vi "Live Capture Functional Stack2.vi"() -> ()   [LabVIEW 2014]
uses:
  subvis/Stack Track.ctl
  subvis/Stack_State.ctl
panel:
  out "error out 2":errorcluster {"code" format="%.0x"}
  out "Count":i32
  in  "Temp":path=path "C:/temp.tmp"
  in  "Frames":i32=100
  in  "HardDisk Record":bool
  in  "Internal Line Interval":dbl
  in  "Slit Width / Lines":sgl=150.0
  in  "Camera Readout Mode":u16(ring)=12 items=["Full Frame"=1, "Slit Scanning"=12]
  in  "Readout Direction":sgl(ring)=1.0 items=["Forward"=1, "Backward"=2]
  in  "Trigger Mode":sgl(ring)=1.0 items=["Normal"=1, "Start "=6]
  in  "Trigger Source":sgl(ring)=2.0 items=["Internal"=1, "External"=2]
  out "Enum":T1
  out "Image":u16[][](graph)
  out "Saving":bool
  in  "AutoIncrement":bool=TRUE
  in  "Path":path=path "C:/Users/spim/Desktop/Craig Cap/temp/a.tiff"
  in  "Frames":i32=100
  out "Frame Index":i32
  out "error out":errorcluster
  in  "stop":bool
  in  "Capture":bool
  out "Total Frames":i32
  out "Elapsed Time":u32
  out "Software FPS":dbl
  out "Camera FPS":dbl
  in  "H Offset":i32 min=0 max=0 step=4
  in  "H Width":i32 min=0 max=2048 step=4
  out "SMD":dbl
  out "SHO":i32
  in  "V Offset":i32 min=0 max=0 step=4
  in  "V Width":i32 min=0 max=2048 step=4
  in  "Binning":u16(ring) items=["1x1"=1, "2x2"=2, "4x4"=4]
  out "SHW":i32
  out "SVO":i32
  out "SVW":i32
  in  "Scan Mode":dbl min=0.0 max=2.0 step=1.0
  in  "Exposure":dbl min=0.0 max=10.000004210526315 step=1e-08
  out "EXP":dbl
  out "Camera Model":string
  out "Camera Version":string
  out "Camera Serial":string
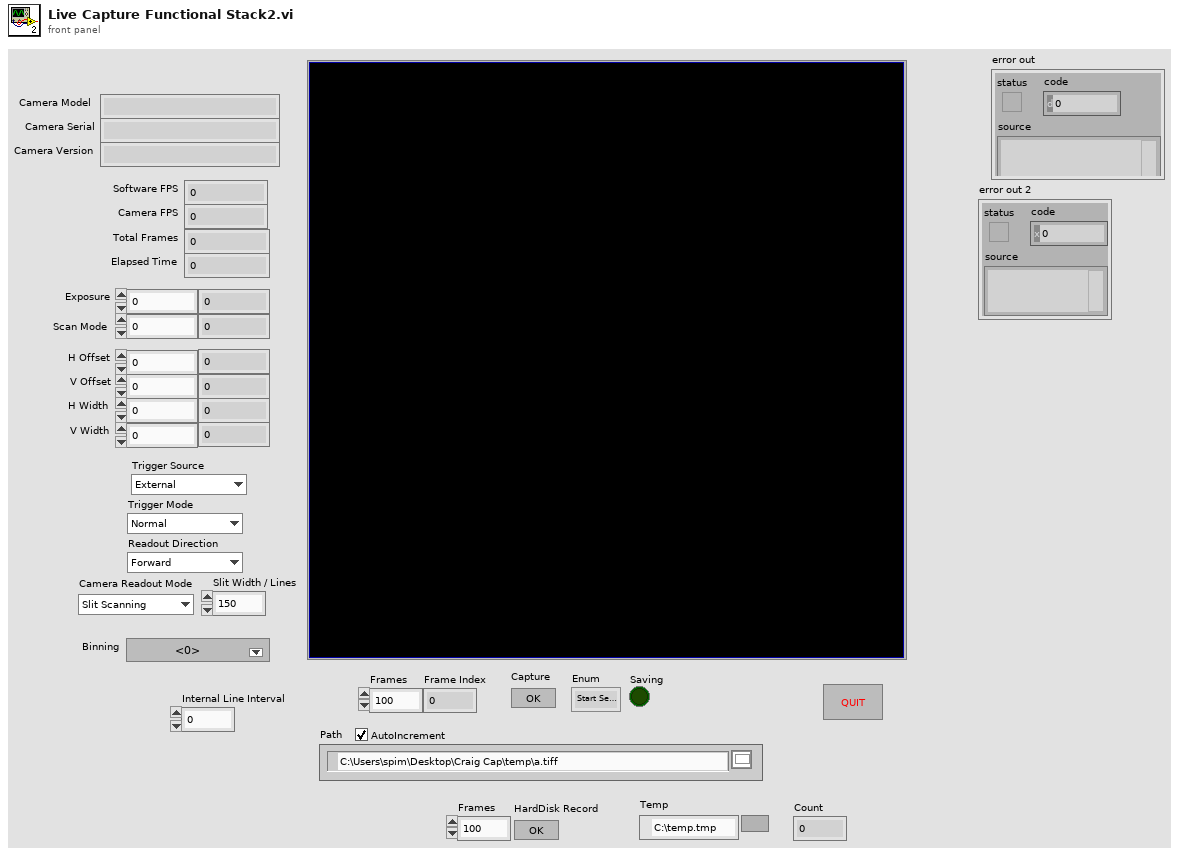
[diagram p1: front panel]
types:
  T1 = typedef "Stack Track.ctl" = enum16{"Start Sequence", "Read Disk", "Idle", "STOP", "Collecting", "End"}
  T2 = enum8{"Enabled", "Disabled", "Disabled and Grayed Out"}
  T3 = typedef "Stack_State.ctl" = cluster{"Enum":T1, "Stack Number":i32}
  T4 = cluster{"Model":string, "Camera ID":string, "Firmware":string}
  T5 = cluster{"Value":i32, "Minimum":i32, "Maximum":i32, "Increment":i32}
  T6 = cluster{"height":u32, "width":u32, "datatype":u32}
  T7 = cluster{"H Offset":i32, "V Offset":i32, "H Width":i32, "V Width":i32}
  T8 = typedef "Image Type" = u32
  T9 = typedef "IMAQ Image.ctl" = refnum<image>
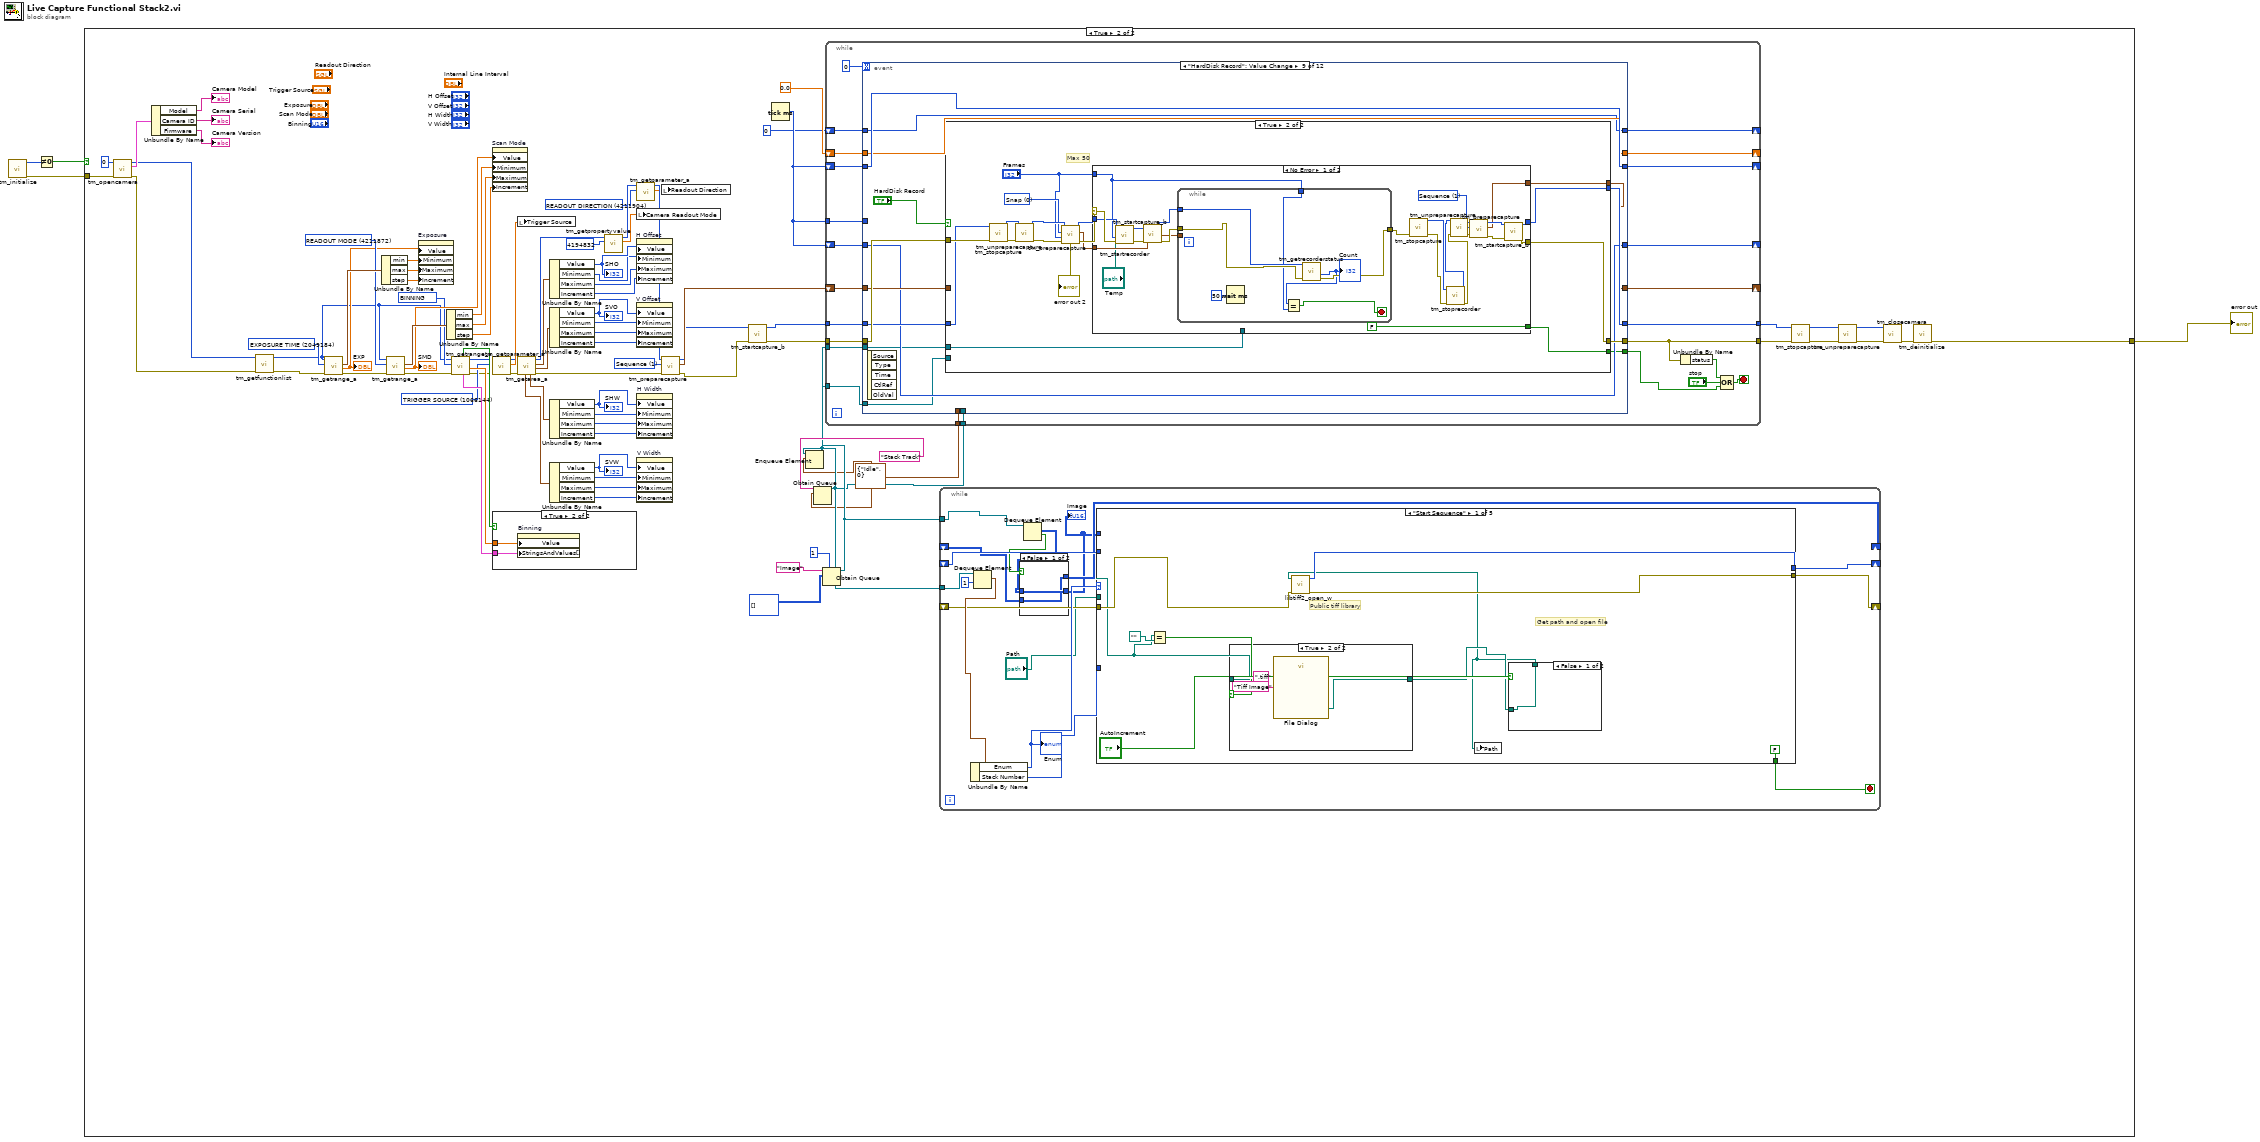
[diagram p0: block diagram]
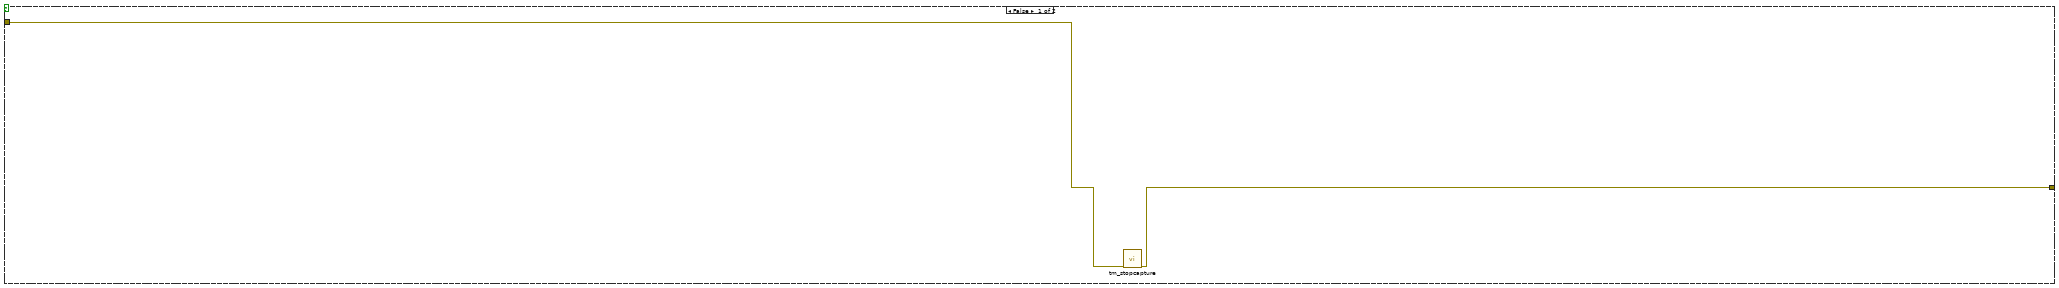
[diagram p2: hidden frame]
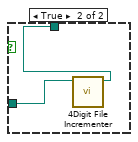
[diagram p5: hidden frame]
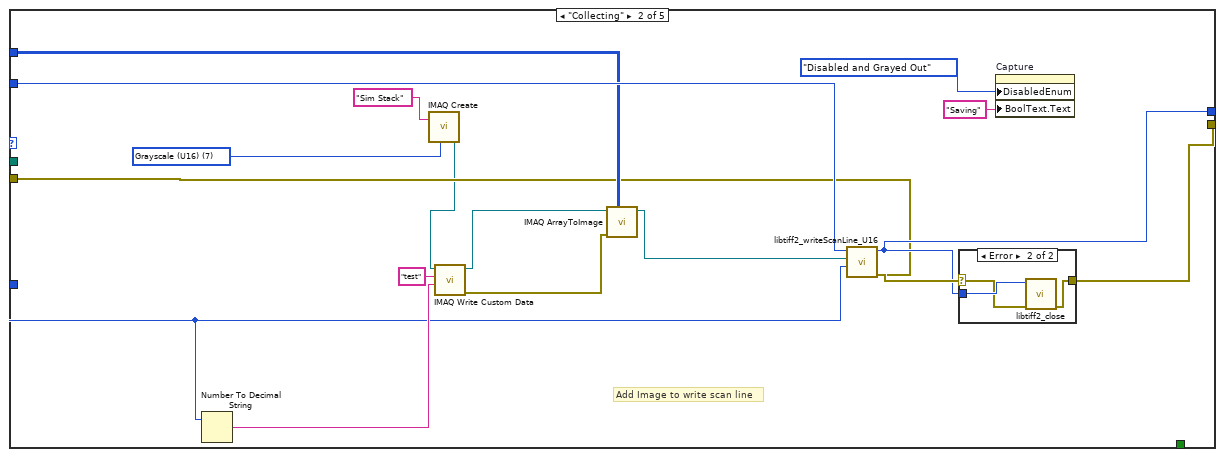
[diagram p6: hidden frame]
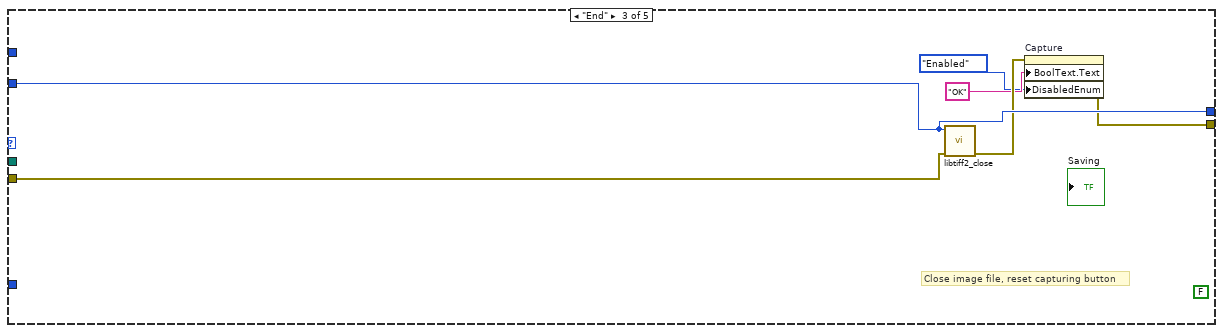
[diagram p8: hidden frame]
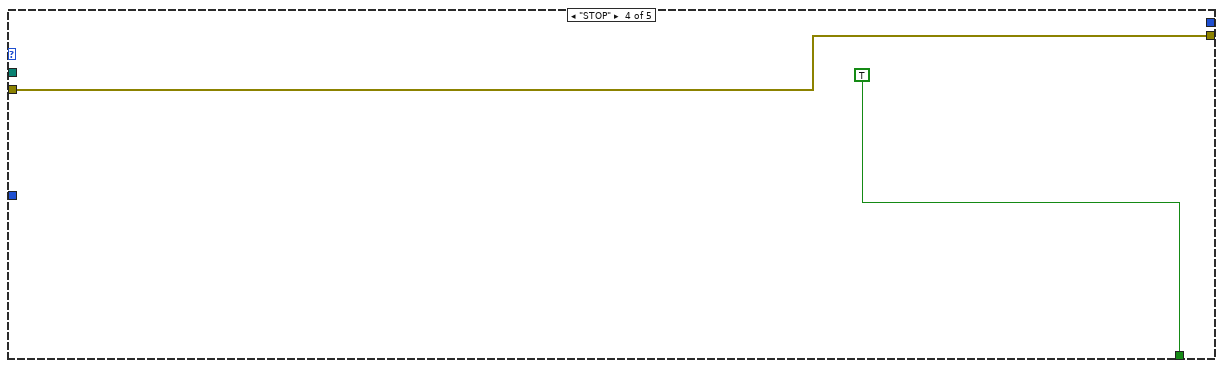
[diagram p9: hidden frame]
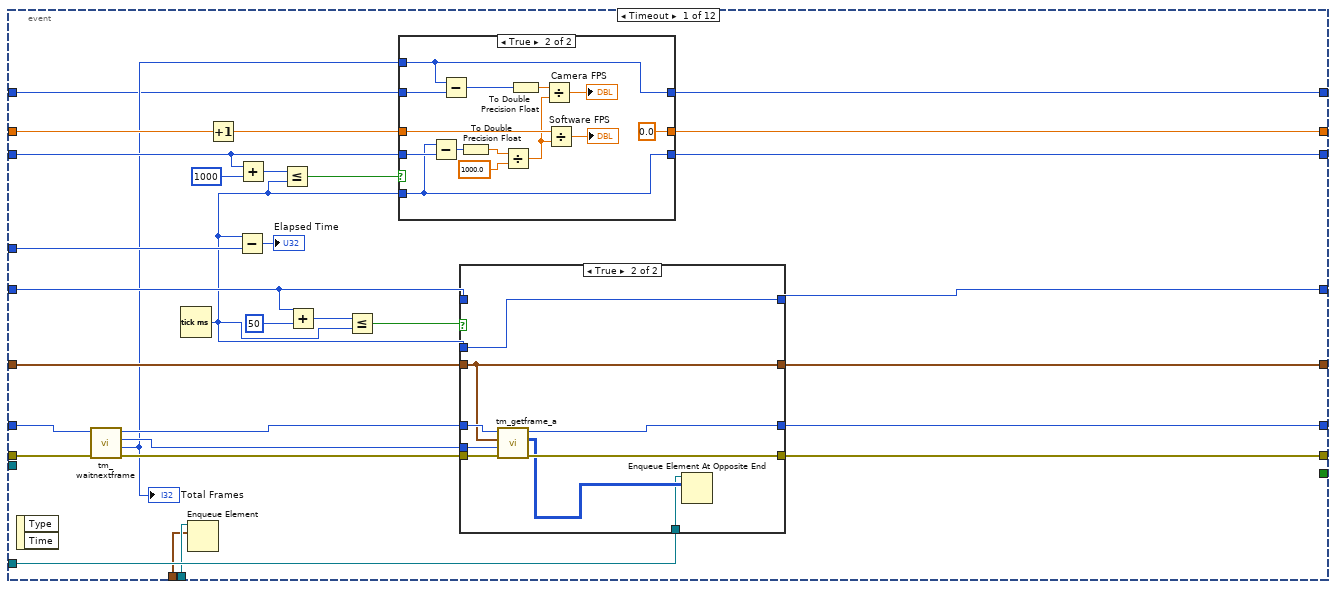
[diagram p12: hidden frame]
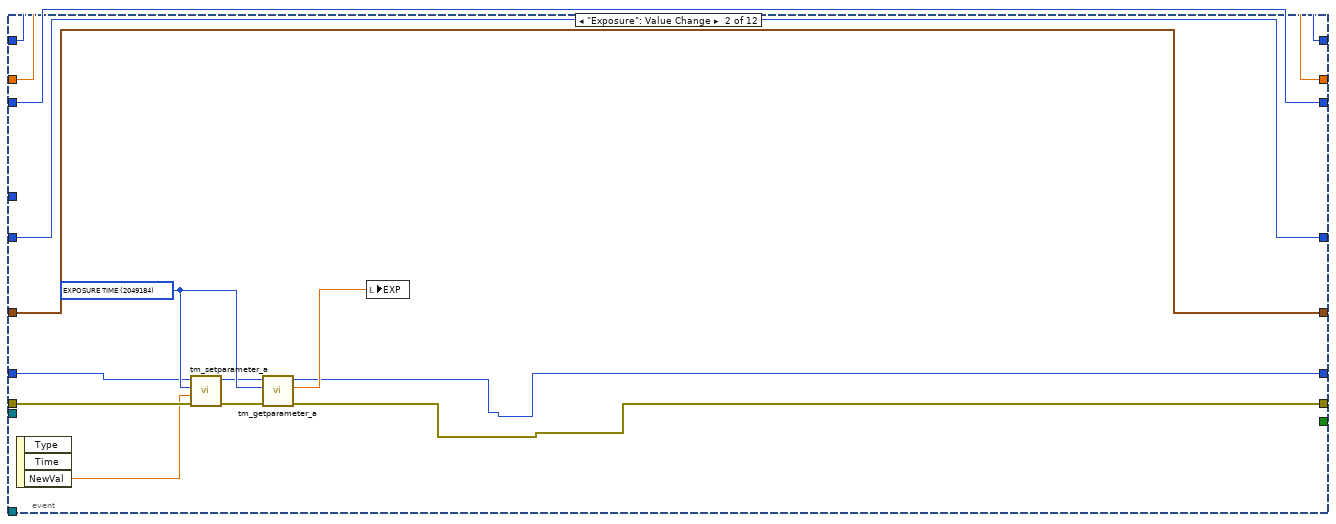
[diagram p15: hidden frame]
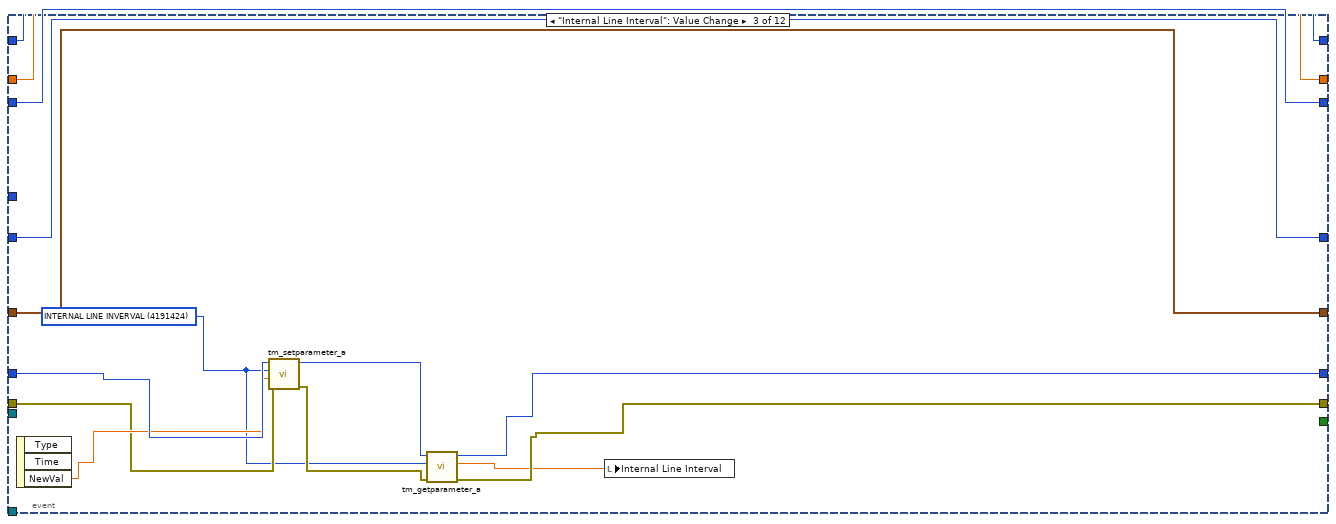
[diagram p16: hidden frame]
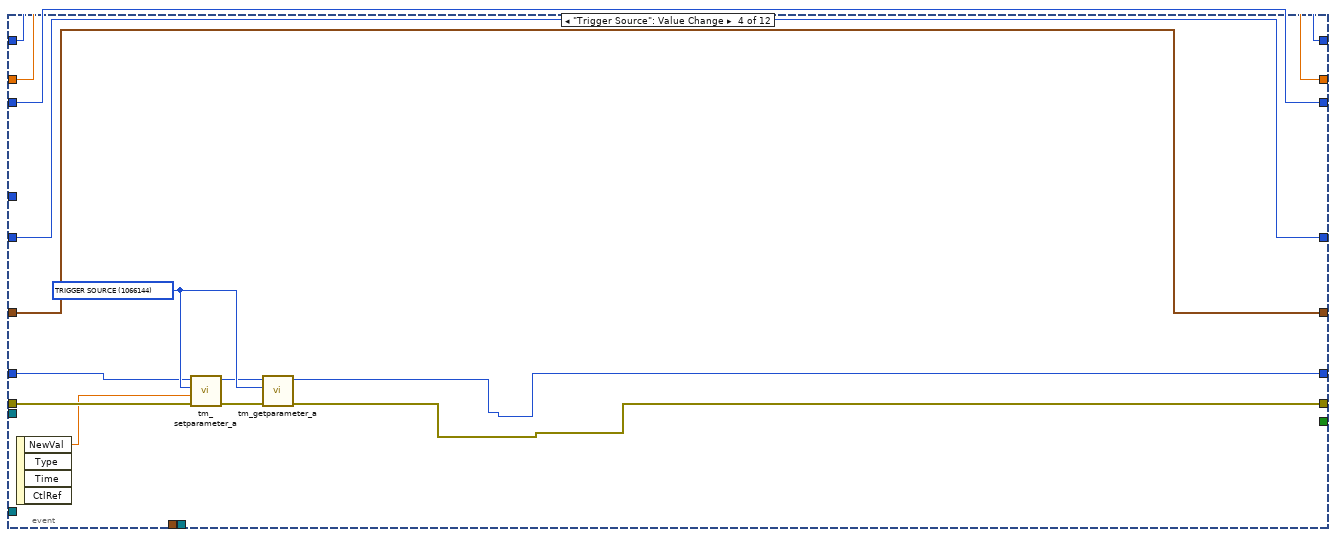
[diagram p17: hidden frame]
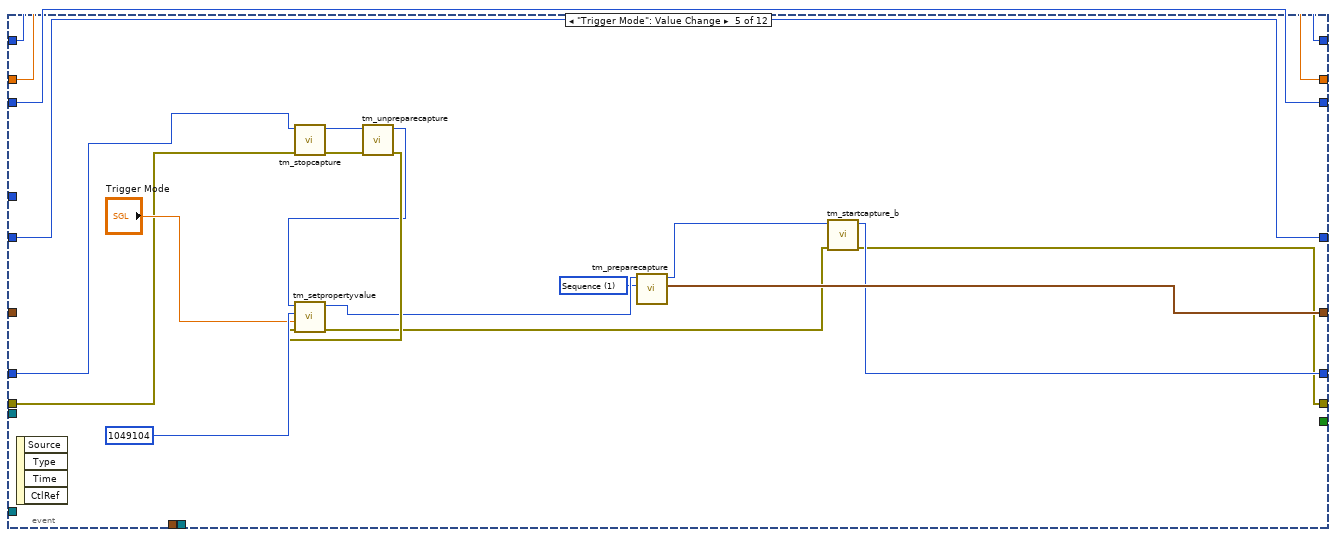
[diagram p18: hidden frame]
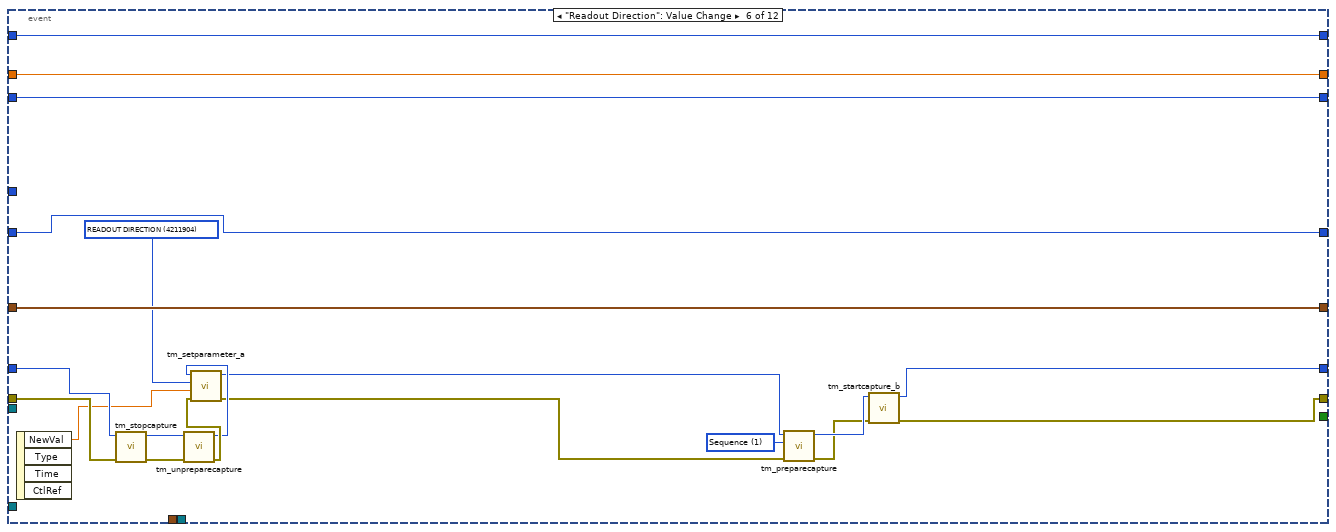
[diagram p19: hidden frame]
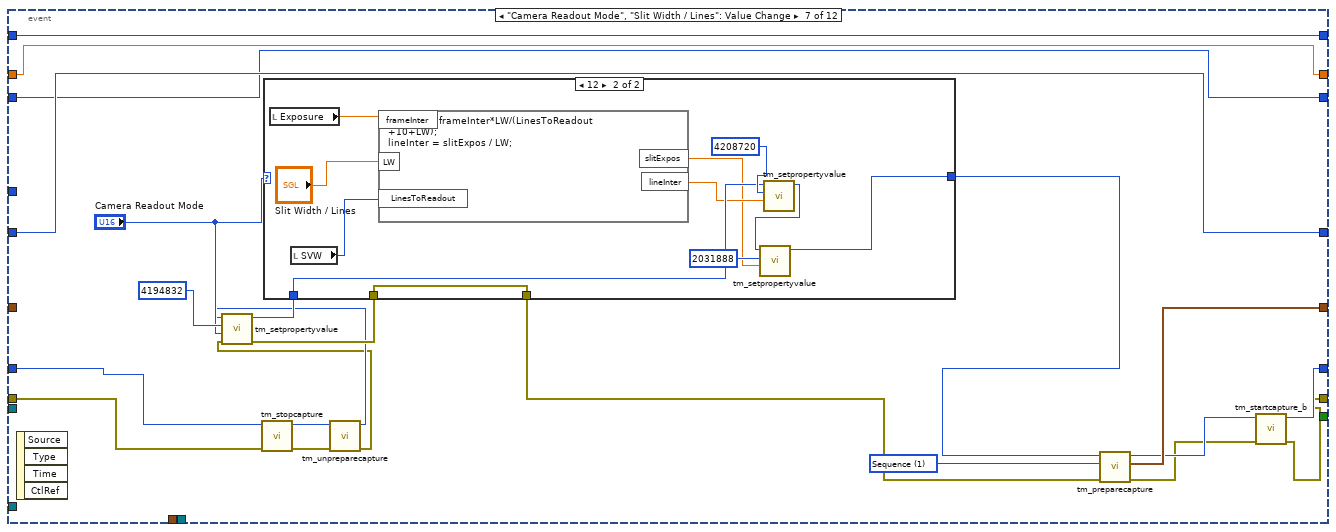
[diagram p20: hidden frame]
diagram:
  n1 = call <userlib>:"tm_initialize.vi"() -> ("error out"=w2:errorcluster, "Number Of Cameras"=w1:u32)  [unwired: 8 in, 2 out]
  n2 = Not Equal To 0?(x=w1) -> (x != 0?=w4:bool)
  n3 = case shown="True" w4 {
    tunnel: [w5 w89] -> w3
    tunnel: w2 -> [w6 w92]
    frame False {
      n4 = call <userlib>:"tm_stopcapture.vi"("error in (no error)"=w6) -> ("error out"=w5:errorcluster)  [unwired: 9 in, 1 out]
    }
    frame True {
      w11 = u32 4211904 items=["SENSOR MODE"=4212128, "CCD MODE"=4212384, "READOUT MODE"=4211872, "ACTIVE VIEW INDEX"=4343136, "BITS PER CHANNEL"=4342976, "IMAGE PIXEL TYPE"=4343296, "BINNING"=4215968, "EXPOSURE TIME"=2049184, "CONTRAST GAIN"=3163312, "CONTRAST OFFSET"=3163328, "LIGHT MODE"=2114720, "SENSITIVITY"=2114992, "PHOTON IMAGING MODE"=2115200, "HIGH DYNAMIC RANGE MODE"=3163360, "WHITE BALANCE"=3163568, "TEMPERATURE"=2115232, "TEMPERATURE TARGET"=2115264, "SENSOR COOLER FAN"=2115296, "LINEBUNDLE HEIGHT"=4212192, "MECHANICAL SHUTTER"=2115488, "BACK FOCUS POSITION"=8422304, "TRIGGER CONNECTOR"=1066432, "TRIGGER SOURCE"=1066144, "OUTPUT TRIGGER SOURCE"=1852576, "TRIGGER GLOBAL EXPOSURE"=2049680, "FIRST TRIGGER BEHAVIOR"=2049696, "CHANNEL SYNC"=1852352, "READOUT DIRECTION"=4211904, "PRE HSYNC COUNT"=1852704] ("Parameter")
      w21 = u32 1066144 items=["SENSOR MODE"=4212128, "CCD MODE"=4212384, "READOUT MODE"=4211872, "ACTIVE VIEW INDEX"=4343136, "BITS PER CHANNEL"=4342976, "IMAGE PIXEL TYPE"=4343296, "BINNING"=4215968, "EXPOSURE TIME"=2049184, "CONTRAST GAIN"=3163312, "CONTRAST OFFSET"=3163328, "LIGHT MODE"=2114720, "SENSITIVITY"=2114992, "PHOTON IMAGING MODE"=2115200, "HIGH DYNAMIC RANGE MODE"=3163360, "WHITE BALANCE"=3163568, "TEMPERATURE"=2115232, "TEMPERATURE TARGET"=2115264, "SENSOR COOLER FAN"=2115296, "LINEBUNDLE HEIGHT"=4212192, "MECHANICAL SHUTTER"=2115488, "BACK FOCUS POSITION"=8422304, "TRIGGER CONNECTOR"=1066432, "TRIGGER SOURCE"=1066144, "OUTPUT TRIGGER SOURCE"=1852576, "TRIGGER GLOBAL EXPOSURE"=2049680, "FIRST TRIGGER BEHAVIOR"=2049696, "CHANNEL SYNC"=1852352, "READOUT DIRECTION"=4211904, "PRE HSYNC COUNT"=1852704] ("Parameter")
      w28 = T3 {"Enum"=enum."Idle", "Stack Number"=0} ("input cluster")
      w35 = u32 2049184 items=["BINNING"=4215968, "BITS PER CHANNEL"=4342976, "ACTIVE VIEW INDEX"=4343136, "CCD MODE"=4212384, "SENSOR MODE"=4212128, "READOUT MODE"=4211872, "EXPOSURE TIME"=2049184, "CONTRAST GAIN"=3163312, "CONTRAST OFFSET"=3163328, "LIGHT MODE"=2114720, "SENSITIVITY"=2114992, "WHITE BALANCE"=3163568, "PHOTON IMAGING MODE"=2115200, "HIGH DYNAMIC RANGE MODE"=3163360, "TRIGGER SOURCE"=1066144, "TRIGGER ACTIVE"=1066160, "TRIGGER MODE"=1066400, "TRIGGER POLARITY"=1066416, "TRIGGER GLOBAL EXPOSURE"=2049680, "FIRST TRIGGER BEHAVIOR"=2049696, "TRIGGER TIMES"=1066448, "OUTPUT TRIGGER POLARITY"=1852592, "OUTPUT TRIGGER DELAY"=1852624, "OUTPUT TRIGGER PERIOD"=1852640, "TEMPERATURE"=2115232, "TEMPERATURE TARGET"=2115264, "SENSOR COOLER FAN"=2115296, "MECHANICAL SHUTTER"=2115488, "BACK FOCUS POSITION"=8422304, "FRAMEBUNDLE MODE"=4346784, "FRAMEBUNDLE NUMBER"=4346800, "LINEBUNDLE HEIGHT"=4212192, "TRIGGER CONNECTOR"=1066432, "IMAGE PIXEL TYPE"=4343296, "OUTPUT TRIGGER KIND"=1852656, "READOUT DIRECTION"=4211904, "CHANNEL SYNC"=1852352] ("Parameter")
      w36 = u32 4211872 items=["BINNING"=4215968, "BITS PER CHANNEL"=4342976, "ACTIVE VIEW INDEX"=4343136, "CCD MODE"=4212384, "SENSOR MODE"=4212128, "READOUT MODE"=4211872, "EXPOSURE TIME"=2049184, "CONTRAST GAIN"=3163312, "CONTRAST OFFSET"=3163328, "LIGHT MODE"=2114720, "SENSITIVITY"=2114992, "WHITE BALANCE"=3163568, "PHOTON IMAGING MODE"=2115200, "HIGH DYNAMIC RANGE MODE"=3163360, "TRIGGER SOURCE"=1066144, "TRIGGER ACTIVE"=1066160, "TRIGGER MODE"=1066400, "TRIGGER POLARITY"=1066416, "TRIGGER GLOBAL EXPOSURE"=2049680, "FIRST TRIGGER BEHAVIOR"=2049696, "TRIGGER TIMES"=1066448, "OUTPUT TRIGGER POLARITY"=1852592, "OUTPUT TRIGGER DELAY"=1852624, "OUTPUT TRIGGER PERIOD"=1852640, "TEMPERATURE"=2115232, "TEMPERATURE TARGET"=2115264, "SENSOR COOLER FAN"=2115296, "MECHANICAL SHUTTER"=2115488, "BACK FOCUS POSITION"=8422304, "FRAMEBUNDLE MODE"=4346784, "FRAMEBUNDLE NUMBER"=4346800, "LINEBUNDLE HEIGHT"=4212192, "TRIGGER CONNECTOR"=1066432, "IMAGE PIXEL TYPE"=4343296, "OUTPUT TRIGGER KIND"=1852656, "READOUT DIRECTION"=4211904, "CHANNEL SYNC"=1852352] ("Parameter")
      w37 = u32 4215968 items=["BINNING"=4215968, "BITS PER CHANNEL"=4342976, "ACTIVE VIEW INDEX"=4343136, "CCD MODE"=4212384, "SENSOR MODE"=4212128, "READOUT MODE"=4211872, "EXPOSURE TIME"=2049184, "CONTRAST GAIN"=3163312, "CONTRAST OFFSET"=3163328, "LIGHT MODE"=2114720, "SENSITIVITY"=2114992, "WHITE BALANCE"=3163568, "PHOTON IMAGING MODE"=2115200, "HIGH DYNAMIC RANGE MODE"=3163360, "TRIGGER SOURCE"=1066144, "TRIGGER ACTIVE"=1066160, "TRIGGER MODE"=1066400, "TRIGGER POLARITY"=1066416, "TRIGGER GLOBAL EXPOSURE"=2049680, "FIRST TRIGGER BEHAVIOR"=2049696, "TRIGGER TIMES"=1066448, "OUTPUT TRIGGER POLARITY"=1852592, "OUTPUT TRIGGER DELAY"=1852624, "OUTPUT TRIGGER PERIOD"=1852640, "TEMPERATURE"=2115232, "TEMPERATURE TARGET"=2115264, "SENSOR COOLER FAN"=2115296, "MECHANICAL SHUTTER"=2115488, "BACK FOCUS POSITION"=8422304, "FRAMEBUNDLE MODE"=4346784, "FRAMEBUNDLE NUMBER"=4346800, "LINEBUNDLE HEIGHT"=4212192, "TRIGGER CONNECTOR"=1066432, "IMAGE PIXEL TYPE"=4343296, "OUTPUT TRIGGER KIND"=1852656, "READOUT DIRECTION"=4211904, "CHANNEL SYNC"=1852352] ("Parameter")
      w87 = 1 items=["Snap", "Sequence"] ("Capture mode")
      n5 = call <userlib>:"tm_opencamera.vi"("error in (no error)"=w92, "Camera Index"=u32 0) -> ("error out"=w25:errorcluster, "Camera Details"=w49:T4, "Handle out"=w9:u32)  [unwired: 7 in]
      n6 = Unbundle By Name(w49) -> ("Model"=→"Camera Model":string, "Camera ID"=→"Camera Serial":string, "Firmware"=→"Camera Version":string)
      n7 = call <userlib>:"tm_getfunctionlist.vi"("error in (no error)"=w25, "Handle in"=w9) -> ("error out"=w24:errorcluster, "Handle out"=w26:u32)  [unwired: 7 in, 1 out]
      n8 = call <userlib>:"tm_getrange_a.vi"("error in (no error)"=w24, "Parameter"=w35, "Handle in"=w26) -> ("error out"=w44:errorcluster, "default"=w27:dbl, "Range"=w45:cluster{"min":dbl, "max":dbl, "step":dbl})  [unwired: 2 in, 4 out]
      "EXP" <- w27
      n9 = Unbundle By Name(w45) -> ("min"=w82:dbl, "max"=w81:dbl, "step"=w80:dbl)
      n10 = call <userlib>:"tm_getrange_a.vi"("error in (no error)"=w44, "Parameter"=w36, "Handle in"=w26) -> ("error out"=w41:errorcluster, "default"=w42:dbl, "Range"=w43:cluster{"min":dbl, "max":dbl, "step":dbl})  [unwired: 2 in, 4 out]
      "SMD" <- w42
      n11 = property on="Exposure" class="DigNum (strict)"("Value"=w27, "Minimum"=w82, "Maximum"=w81, "Increment"=w80) -> ()  [unwired: 2 in, 2 out]
      n12 = Unbundle By Name(w43) -> ("min"=w79:dbl, "max"=w78:dbl, "step"=w77:dbl)
      n13 = call <userlib>:"tm_getrange_a.vi"("error in (no error)"=w41, "Parameter"=w37, "Handle in"=w26) -> ("error out"=w18:errorcluster, "default"=w39:dbl, "Handle out"=w20:u32, "Value Names"=w38:cluster{"Name":string, "Value":dbl}[], "Writable"=w40:bool)  [unwired: 2 in, 2 out]
      n14 = property on="Scan Mode" class="DigNum (strict)"("Value"=w42, "Minimum"=w79, "Maximum"=w78, "Increment"=w77) -> ()  [unwired: 2 in, 2 out]
      n15 = call <userlib>:"tm_getparameter_a.vi"("error in (no error)"=w18, "Parameter"=w21, "Handle in"=w20) -> ("error out"=w17:errorcluster, "Value out"=w22:dbl, "Handle out"=w19:u32)  [unwired: 6 in]
      n16 = case shown="True" w40 {
        tunnel: w38 -> [_ w162]
        tunnel: w39 -> [_ w161]
        frame False {
        }
        frame True {
          n17 = property on="Binning" class="Ring (strict)"("Value"=w161, "StringsAndValues[]"=w162) -> ()  [unwired: 2 in, 2 out]
        }
      }
      n18 = local write "Trigger Source"(w22) -> ()
      n19 = call <userlib>:"tm_getarea_a.vi"("error in (no error)"=w17, "Handle in"=w19) -> ("error out"=w23:errorcluster, "V Offset"=w76:T5, "H Offset"=w55:T5, "Handle out"=w14:u32, "H Width"=w75:T5, "V Width"=w74:T5)  [unwired: 4 in]
      n20 = Unbundle By Name(w55) -> ("Value"=w54:i32, "Minimum"=w53:i32, "Maximum"=w52:i32, "Increment"=w51:i32)
      "SHO" <- w54
      n21 = Unbundle By Name(w76) -> ("Value"=w64:i32, "Minimum"=w73:i32, "Maximum"=w72:i32, "Increment"=w71:i32)
      "SVO" <- w64
      n22 = Unbundle By Name(w75) -> ("Value"=w63:i32, "Minimum"=w70:i32, "Maximum"=w69:i32, "Increment"=w68:i32)
      "SHW" <- w63
      n23 = Unbundle By Name(w74) -> ("Value"=w62:i32, "Minimum"=w67:i32, "Maximum"=w66:i32, "Increment"=w65:i32)
      "SVW" <- w62
      n24 = call <userlib>:"tm_getpropertyvalue.vi"("Property ID"=u32 4194832, "Handle in"=w14) -> ("Value in"=w15:sgl, "Handle out"=w13:u32)  [unwired: 7 in, 1 out]
      n25 = call <userlib>:"tm_getparameter_a.vi"("Parameter"=w11, "Handle in"=w13) -> ("Value out"=w10:dbl, "Handle out"=w12:u32)  [unwired: 7 in, 1 out]
      n26 = local write "Camera Readout Mode"(w15) -> ()
      n27 = property on="H Offset" class="DigNum (strict)"("Value"=w54, "Minimum"=w53, "Maximum"=w52, "Increment"=w51) -> ()  [unwired: 2 in, 2 out]
      n28 = property on="V Offset" class="DigNum (strict)"("Value"=w64, "Minimum"=w73, "Maximum"=w72, "Increment"=w71) -> ()  [unwired: 2 in, 2 out]
      n29 = property on="H Width" class="DigNum (strict)"("Value"=w63, "Minimum"=w70, "Maximum"=w69, "Increment"=w68) -> ()  [unwired: 2 in, 2 out]
      n30 = property on="V Width" class="DigNum (strict)"("Value"=w62, "Minimum"=w67, "Maximum"=w66, "Increment"=w65) -> ()  [unwired: 2 in, 2 out]
      n31 = local write "Readout Direction"(w10) -> ()
      n32 = call <userlib>:"tm_preparecapture.vi"("error in (no error)"=w23, "Capture mode"=w87, "Handle in"=w12) -> ("error out"=w7:errorcluster, "Buffer Info"=w84:T6, "Handle out"=w8:u32)  [unwired: 5 in, 1 out]
      n33 = call <userlib>:"tm_startcapture_b.vi"("error in (no error)"=w7, "Handle in"=w8) -> ("error out"=w86:errorcluster, "Handle out"=w85:u32)  [unwired: 8 in]
      n34 = Tick Count (ms)() -> (millisecond timer value=w83:u32)
      n35 = Obtain Queue(name (unnamed)="Stack Track", element data type=w28) -> (queue out=w29:refnum<queue>)  [unwired: 3 in, 2 out]
      n36 = Enqueue Element(queue=w29, element=w28) -> ()  [unwired: 2 in, 3 out]
      n37 = Obtain Queue(max queue size (-1, unlimited)=1, name (unnamed)="Image", element data type=u16[][] []) -> (queue out=w30:refnum<queue>)  [unwired: 2 in, 2 out]
      n38 = while {
        tunnel: w86 -> [w175]
        tunnel: [w173] -> w61
        tunnel: [w172] -> w60
        shift-right: [w182] -> _
        shift-left: w83 -> [w180]
        shift-right: [w183] -> _
        shift-left: 0.0 -> [w181]
        shift-right: [w174] -> _
        shift-left: w83 -> [w178]
        tunnel: w85 -> [w176]
        tunnel: w83 -> [w179]
        shift-right: [w171] -> _
        shift-left: w84 -> [w177]
        shift-right: [w168] -> _
        shift-left: 0 -> [w169]
        tunnel: w30 -> [w166]
        tunnel: w29 -> [w167]
        tunnel: w29 -> [w165]
        tunnel: w28 -> [w164]
        stop <- w184 stop-if-true
        n39 = event shown="[8] \"HardDisk Record\": Value Change" {
          selector: _ -> [_ _ _ _ _ _ _ _ _ _ _ _]
          dyn-events: _ -> [_ _ _ _ _ _ _ _ _ _ _ _]
          timeout: 0 -> [_ _ _ _ _ _ _ _ _ _ _ _]
          tunnel: [w195 w259 w273 w286 w305 w325 w347 w374 w475 w566 w602 w647] -> w183
          tunnel: [w194 w260 w274 w287 w306 w326 w348 w375 w476 w567 w603 w648] -> w182
          tunnel: w181 -> [w206 w259 w273 w286 w305 w325 w347 w374 w475 w566 w602 w647]
          tunnel: w180 -> [w197 w260 w274 w287 w306 w326 w348 w375 w476 w567 w603 w648]
          tunnel: w179 -> [w202 _ _ _ _ _ _ _ _ _ _ _]
          tunnel: w178 -> [w207 w261 w275 w288 w307 w327 w349 w370 w471 w568 w610 w655]
          tunnel: w177 -> [w201 w258 w272 w285 _ w324 _ w371 w472 _ _ _]
          tunnel: w176 -> [w209 w253 w267 w281 w299 w318 w340 w378 w479 w563 w579 w617]
          tunnel: w175 -> [w208 w255 w263 w282 w298 w321 w339 w379 w480 w562 w578 w616]
          tunnel: [w205 w261 w275 w288 w307 w327 w349 w370 w471 w568 w610 w655] -> w174
          tunnel: [w204 w249 w270 w278 w290 w311 w330 w376 w477 w557 w605 w650] -> w173
          tunnel: [w203 w248 w269 w277 w289 w310 w328 w377 w478 w558 w606 w651] -> w172
          tunnel: [w200 w258 w272 w285 w293 w324 w335 w372 w473 w556 w604 w649] -> w171
          tunnel: w169 -> [w192 w257 w271 w284 w304 w323 w346 w373 w474 w555 w575 w611]
          tunnel: [w191 w257 w271 w284 w304 w323 w346 w373 w474 w555 w575 w611] -> w168
          tunnel: w166 -> [w189 _ _ _ _ _ _ w368 w469 _ _ _]
          tunnel: w167 -> [_ _ _ _ _ _ _ w369 w470 _ _ _]
          tunnel: w165 -> [w188 _ _ _ _ _ _ _ _ _ _ _]
          tunnel: w164 -> [w187 _ _ _ _ _ _ _ _ _ _ _]
          tunnel: [_ _ _ _ _ _ _ w367 w468 _ _ _] -> w163
          event Timeout {
            n40 = event-data() -> ()  [unwired: 1 in, 2 out]
            n41 = call <userlib>:"tm_waitnextframe.vi"("error in (no error)"=w208, "Handle in"=w209) -> ("error out"=w212:errorcluster, "Frame Count"=w193:i32, "Frame Index"=w211:i32, "Handle out"=w213:u32)  [unwired: 6 in]
            "Total Frames" <- w193
            n42 = Tick Count (ms)() -> (millisecond timer value=w199:u32)
            n43 = Enqueue Element(queue=w188, element=w187) -> ()  [unwired: 2 in, 3 out]
            n44 = Increment(x=w206) -> (x+1=w196:dbl)
            n45 = Subtract(x=w199, y=w202) -> (x-y=→"Elapsed Time":u32)
            n46 = Add(x=w197, y=u32 1000) -> (x+y=w217:u32)
            n47 = Less Or Equal?(x=w217, y=w199) -> (x <= y?=w198:bool)
            n48 = Add(x=w207, y=u32 50) -> (x+y=w215:u32)
            n49 = Less Or Equal?(x=w215, y=w199) -> (x <= y?=w190:bool)
            n50 = case shown="True" w198 {
              tunnel: w197 -> [w220 w229]
              tunnel: [w220 w226] -> w194
              tunnel: w196 -> [w219 w232]
              tunnel: w199 -> [_ w226]
              tunnel: [w219 0.0] -> w195
              tunnel: w193 -> [_ w221]
              tunnel: w192 -> [w218 w224]
              tunnel: [w218 w221] -> w191
              frame False {
              }
              frame True {
                n51 = Subtract(x=w226, y=w229) -> (x-y=w228:u32)
                n52 = Subtract(x=w221, y=w224) -> (x-y=w222:i32)
                n53 = To Double Precision Float(number=w228) -> (double precision float=w234:dbl)
                n54 = Divide(x=w234, y=1000.0) -> (x/y=w225:dbl)
                n55 = To Double Precision Float(number=w222) -> (double precision float=w223:dbl)
                n56 = Divide(x=w223, y=w225) -> (x/y=→"Camera FPS":dbl)
                n57 = Divide(x=w232, y=w225) -> (x/y=→"Software FPS":dbl)
              }
            }
            n58 = case shown="True" w190 {
              tunnel: w207 -> [w238 _]
              tunnel: w199 -> [_ w247]
              tunnel: [w238 w247] -> w205
              tunnel: w213 -> [w237 w246]
              tunnel: w201 -> [w235 w241]
              tunnel: w212 -> [w236 w245]
              tunnel: [w237 w244] -> w204
              tunnel: [w236 w243] -> w203
              tunnel: w211 -> [_ w242]
              tunnel: [w235 w241] -> w200
              tunnel: w189 -> [_ w239]
              frame False {
              }
              frame True {
                n59 = call <userlib>:"tm_getframe_a.vi"("error in (no error)"=w245, "Frame Index"=w242, "Buffer Info"=w241, "Handle in"=w246) -> ("error out"=w243:errorcluster, "Data 16"=w240:u16[][], "Handle out"=w244:u32)  [unwired: 3 in, 2 out]
                n60 = Enqueue Element At Opposite End(queue=w239, element=w240) -> ()  [unwired: 2 in, 3 out]
              }
            }
          }
          event "Exposure": Value Change {
            w256 = u32 2049184 items=["SENSOR MODE"=4212128, "CCD MODE"=4212384, "READOUT MODE"=4211872, "ACTIVE VIEW INDEX"=4343136, "BITS PER CHANNEL"=4342976, "IMAGE PIXEL TYPE"=4343296, "BINNING"=4215968, "EXPOSURE TIME"=2049184, "CONTRAST GAIN"=3163312, "CONTRAST OFFSET"=3163328, "LIGHT MODE"=2114720, "SENSITIVITY"=2114992, "PHOTON IMAGING MODE"=2115200, "HIGH DYNAMIC RANGE MODE"=3163360, "WHITE BALANCE"=3163568, "TEMPERATURE"=2115232, "TEMPERATURE TARGET"=2115264, "SENSOR COOLER FAN"=2115296, "LINEBUNDLE HEIGHT"=4212192, "MECHANICAL SHUTTER"=2115488, "BACK FOCUS POSITION"=8422304, "TRIGGER CONNECTOR"=1066432, "TRIGGER SOURCE"=1066144, "OUTPUT TRIGGER SOURCE"=1852576, "TRIGGER GLOBAL EXPOSURE"=2049680, "FIRST TRIGGER BEHAVIOR"=2049696, "CHANNEL SYNC"=1852352, "READOUT DIRECTION"=4211904, "PRE HSYNC COUNT"=1852704] ("Parameter")
            n61 = event-data() -> ("NewVal"=w254:dbl)  [unwired: 1 in, 2 out]
            n62 = call <userlib>:"tm_setparameter_a.vi"("error in (no error)"=w255, "Value in"=w254, "Parameter"=w256, "Handle in"=w253) -> ("error out"=w252:errorcluster, "Handle out"=w251:u32)  [unwired: 6 in]
            n63 = call <userlib>:"tm_getparameter_a.vi"("error in (no error)"=w252, "Parameter"=w256, "Handle in"=w251) -> ("error out"=w248:errorcluster, "Value out"=w250:dbl, "Handle out"=w249:u32)  [unwired: 6 in]
            n64 = local write "EXP"(w250) -> ()
          }
          event "Internal Line Interval": Value Change {
            w262 = u32 4191424 items=["SENSOR MODE"=4212128, "CCD MODE"=4212384, "READOUT MODE"=4211872, "ACTIVE VIEW INDEX"=4343136, "BITS PER CHANNEL"=4342976, "IMAGE PIXEL TYPE"=4343296, "BINNING"=4215968, "EXPOSURE TIME"=2049184, "CONTRAST GAIN"=3163312, "CONTRAST OFFSET"=3163328, "LIGHT MODE"=2114720, "SENSITIVITY"=2114992, "PHOTON IMAGING MODE"=2115200, "HIGH DYNAMIC RANGE MODE"=3163360, "WHITE BALANCE"=3163568, "TEMPERATURE"=2115232, "TEMPERATURE TARGET"=2115264, "SENSOR COOLER FAN"=2115296, "LINEBUNDLE HEIGHT"=4212192, "MECHANICAL SHUTTER"=2115488, "BACK FOCUS POSITION"=8422304, "TRIGGER CONNECTOR"=1066432, "TRIGGER SOURCE"=1066144, "OUTPUT TRIGGER SOURCE"=1852576, "TRIGGER GLOBAL EXPOSURE"=2049680, "FIRST TRIGGER BEHAVIOR"=2049696, "CHANNEL SYNC"=1852352, "READOUT DIRECTION"=4211904, "PRE HSYNC COUNT"=1852704, "INTERNAL LINE SPEED"=4191408, "INTERNAL LINE INVERVAL"=4191424] ("Parameter")
            n65 = event-data() -> ("NewVal"=w266:dbl)  [unwired: 1 in, 2 out]
            n66 = call <userlib>:"tm_setparameter_a.vi"("error in (no error)"=w263, "Value in"=w266, "Parameter"=w262, "Handle in"=w267) -> ("error out"=w264:errorcluster, "Handle out"=w265:u32)  [unwired: 6 in]
            n67 = call <userlib>:"tm_getparameter_a.vi"("error in (no error)"=w264, "Parameter"=w262, "Handle in"=w265) -> ("error out"=w269:errorcluster, "Value out"=w268:dbl, "Handle out"=w270:u32)  [unwired: 6 in]
            n68 = local write "Internal Line Interval"(w268) -> ()
          }
          event "Trigger Source": Value Change {
            w283 = u32 1066144 items=["SENSOR MODE"=4212128, "CCD MODE"=4212384, "READOUT MODE"=4211872, "ACTIVE VIEW INDEX"=4343136, "BITS PER CHANNEL"=4342976, "IMAGE PIXEL TYPE"=4343296, "BINNING"=4215968, "EXPOSURE TIME"=2049184, "CONTRAST GAIN"=3163312, "CONTRAST OFFSET"=3163328, "LIGHT MODE"=2114720, "SENSITIVITY"=2114992, "PHOTON IMAGING MODE"=2115200, "HIGH DYNAMIC RANGE MODE"=3163360, "WHITE BALANCE"=3163568, "TEMPERATURE"=2115232, "TEMPERATURE TARGET"=2115264, "SENSOR COOLER FAN"=2115296, "LINEBUNDLE HEIGHT"=4212192, "MECHANICAL SHUTTER"=2115488, "BACK FOCUS POSITION"=8422304, "TRIGGER CONNECTOR"=1066432, "TRIGGER SOURCE"=1066144, "OUTPUT TRIGGER SOURCE"=1852576, "TRIGGER GLOBAL EXPOSURE"=2049680, "FIRST TRIGGER BEHAVIOR"=2049696, "CHANNEL SYNC"=1852352, "READOUT DIRECTION"=4211904, "PRE HSYNC COUNT"=1852704] ("Parameter")
            n69 = event-data() -> ("NewVal"=w276:sgl)  [unwired: 1 in, 3 out]
            n70 = call <userlib>:"tm_setparameter_a.vi"("error in (no error)"=w282, "Value in"=w276, "Parameter"=w283, "Handle in"=w281) -> ("error out"=w280:errorcluster, "Handle out"=w279:u32)  [unwired: 6 in]
            n71 = call <userlib>:"tm_getparameter_a.vi"("error in (no error)"=w280, "Parameter"=w283, "Handle in"=w279) -> ("error out"=w277:errorcluster, "Handle out"=w278:u32)  [unwired: 6 in, 1 out]
          }
          event "Trigger Mode": Value Change {
            w294 = 1 items=["Snap", "Sequence"] ("Capture mode")
            n72 = event-data() -> ()  [unwired: 1 in, 4 out]
            n73 = call <userlib>:"tm_stopcapture.vi"("error in (no error)"=w298, "Handle in"=w299) -> ("error out"=w301:errorcluster, "Handle out"=w300:u32)  [unwired: 8 in]
            n74 = call <userlib>:"tm_unpreparecapture.vi"("error in (no error)"=w301, "Handle in"=w300) -> ("error out"=w297:errorcluster, "Handle out"=w296:u32)  [unwired: 8 in]
            n75 = call <userlib>:"tm_setpropertyvalue.vi"("error in (no error)"=w297, "Value in"="Trigger Mode", "Property ID"=u32 1049104, "Handle in"=w296) -> ("error out"=w292:errorcluster, "Handle out"=w295:u32)  [unwired: 6 in]
            n76 = call <userlib>:"tm_preparecapture.vi"("Capture mode"=w294, "Handle in"=w295) -> ("Buffer Info"=w293:T6, "Handle out"=w291:u32)  [unwired: 6 in, 2 out]
            n77 = call <userlib>:"tm_startcapture_b.vi"("error in (no error)"=w292, "Handle in"=w291) -> ("error out"=w289:errorcluster, "Handle out"=w290:u32)  [unwired: 8 in]
          }
          event "Readout Direction": Value Change {
            w316 = 1 items=["Snap", "Sequence"] ("Capture mode")
            w309 = u32 4211904 items=["SENSOR MODE"=4212128, "CCD MODE"=4212384, "READOUT MODE"=4211872, "ACTIVE VIEW INDEX"=4343136, "BITS PER CHANNEL"=4342976, "IMAGE PIXEL TYPE"=4343296, "BINNING"=4215968, "EXPOSURE TIME"=2049184, "CONTRAST GAIN"=3163312, "CONTRAST OFFSET"=3163328, "LIGHT MODE"=2114720, "SENSITIVITY"=2114992, "PHOTON IMAGING MODE"=2115200, "HIGH DYNAMIC RANGE MODE"=3163360, "WHITE BALANCE"=3163568, "TEMPERATURE"=2115232, "TEMPERATURE TARGET"=2115264, "SENSOR COOLER FAN"=2115296, "LINEBUNDLE HEIGHT"=4212192, "MECHANICAL SHUTTER"=2115488, "BACK FOCUS POSITION"=8422304, "TRIGGER CONNECTOR"=1066432, "TRIGGER SOURCE"=1066144, "OUTPUT TRIGGER SOURCE"=1852576, "TRIGGER GLOBAL EXPOSURE"=2049680, "FIRST TRIGGER BEHAVIOR"=2049696, "CHANNEL SYNC"=1852352, "READOUT DIRECTION"=4211904, "PRE HSYNC COUNT"=1852704] ("Parameter")
            n78 = event-data() -> ("NewVal"=w308:sgl)  [unwired: 1 in, 3 out]
            n79 = call <userlib>:"tm_stopcapture.vi"("error in (no error)"=w321, "Handle in"=w318) -> ("error out"=w322:errorcluster, "Handle out"=w317:u32)  [unwired: 8 in]
            n80 = call <userlib>:"tm_unpreparecapture.vi"("error in (no error)"=w322, "Handle in"=w317) -> ("error out"=w320:errorcluster, "Handle out"=w319:u32)  [unwired: 8 in]
            n81 = call <userlib>:"tm_setparameter_a.vi"("error in (no error)"=w320, "Value in"=w308, "Parameter"=w309, "Handle in"=w319) -> ("error out"=w313:errorcluster, "Handle out"=w312:u32)  [unwired: 6 in]
            n82 = call <userlib>:"tm_preparecapture.vi"("error in (no error)"=w313, "Capture mode"=w316, "Handle in"=w312) -> ("error out"=w314:errorcluster, "Handle out"=w315:u32)  [unwired: 5 in, 2 out]
            n83 = call <userlib>:"tm_startcapture_b.vi"("error in (no error)"=w314, "Handle in"=w315) -> ("error out"=w310:errorcluster, "Handle out"=w311:u32)  [unwired: 8 in]
          }
          event "Camera Readout Mode", "Slit Width / Lines": Value Change {
            w333 = 1 items=["Snap", "Sequence"] ("Capture mode")
            n84 = event-data() -> ()  [unwired: 1 in, 4 out]
            n85 = call <userlib>:"tm_stopcapture.vi"("error in (no error)"=w339, "Handle in"=w340) -> ("error out"=w341:errorcluster, "Handle out"=w337:u32)  [unwired: 8 in]
            n86 = call <userlib>:"tm_unpreparecapture.vi"("error in (no error)"=w341, "Handle in"=w337) -> ("error out"=w332:errorcluster, "Handle out"=w338:u32)  [unwired: 8 in]
            n87 = call <userlib>:"tm_setpropertyvalue.vi"("error in (no error)"=w332, "Value in"="Camera Readout Mode", "Property ID"=u32 4194832, "Handle in"=w338) -> ("error out"=w342:errorcluster, "Handle out"=w343:u32)  [unwired: 6 in]
            n88 = case shown="12" "Camera Readout Mode" {
              tunnel: w343 -> [w354 w361]
              tunnel: [w353 w356] -> w336
              tunnel: w342 -> [w351 w366]
              tunnel: [w350 w366] -> w334
              frame 1, Default {
                n89 = local read "Exposure"() -> (w352:dbl)
                n90 = call <userlib>:"tm_setpropertyvalue.vi"("error in (no error)"=w351, "Value in"=w352, "Property ID"=u32 2031888, "Handle in"=w354) -> ("error out"=w350:errorcluster, "Handle out"=w353:u32)  [unwired: 6 in]
              }
              frame 12 {
                n91 = local read "Exposure"() -> (w365:dbl)
                n92 = local read "SVW"() -> (w363:i32)
                n93 = formula code="slitExpos=frameInter*LW/(LinesToReadout\n+10+LW);\nlineInter = slitExpos / LW;"("frameInter"=w365, "LW"="Slit Width / Lines", "LinesToReadout"=w363) -> ("slitExpos"=w357:dbl, "lineInter"=w360:dbl)
                n94 = call <userlib>:"tm_setpropertyvalue.vi"("Value in"=w360, "Property ID"=u32 4208720, "Handle in"=w361) -> ("Handle out"=w359:u32)  [unwired: 7 in, 1 out]
                n95 = call <userlib>:"tm_setpropertyvalue.vi"("Value in"=w357, "Property ID"=u32 2031888, "Handle in"=w359) -> ("Handle out"=w356:u32)  [unwired: 7 in, 1 out]
              }
            }
            n96 = call <userlib>:"tm_preparecapture.vi"("error in (no error)"=w334, "Capture mode"=w333, "Handle in"=w336) -> ("error out"=w329:errorcluster, "Buffer Info"=w335:T6, "Handle out"=w331:u32)  [unwired: 5 in, 1 out]
            n97 = call <userlib>:"tm_startcapture_b.vi"("error in (no error)"=w329, "Handle in"=w331) -> ("error out"=w328:errorcluster, "Handle out"=w330:u32)  [unwired: 8 in]
          }
          event "Capture": Value Change {
            n98 = event-data() -> ()  [unwired: 1 in, 5 out]
            n99 = case shown="True" "Capture" {
              tunnel: w379 -> [w383 w406]
              tunnel: w378 -> [w382 w403]
              tunnel: [w383 w384] -> w377
              tunnel: [w382 w386] -> w376
              tunnel: [w381 w385] -> w372
              tunnel: w371 -> [w381 _]
              tunnel: w369 -> [_ w392]
              tunnel: w368 -> [_ w389]
              tunnel: [_ w387] -> w367
              frame False {
              }
              frame True {
                w394 = T3 {"Enum"=enum."Start Sequence", "Stack Number"=0} ("input cluster")
                w400 = 0 items=["Snap", "Sequence"] ("Capture mode")
                # "Max 50"
                n100 = Flush Queue(queue=w392) -> (queue out=w391:refnum<queue>)  [unwired: 1 in, 2 out]
                n101 = call <userlib>:"tm_stopcapture.vi"("error in (no error)"=w406, "Handle in"=w403) -> ("error out"=w405:errorcluster, "Handle out"=w404:u32)  [unwired: 8 in]
                n102 = call <userlib>:"tm_unpreparecapture.vi"("error in (no error)"=w405, "Handle in"=w404) -> ("error out"=w401:errorcluster, "Handle out"=w402:u32)  [unwired: 8 in]
                n103 = call <userlib>:"tm_preparecapture.vi"("error in (no error)"=w401, "Frames"="Frames", "Capture mode"=w400, "Handle in"=w402) -> ("error out"=w399:errorcluster, "Buffer Info"=w397:T6, "Handle out"=w398:u32)  [unwired: 4 in, 1 out]
                n104 = Enqueue Element(queue=w391, element=w394) -> (queue out=w395:refnum<queue>, error out=w390:errorcluster)  [unwired: 2 in, 1 out]
                n105 = Flush Queue(queue=w389, error in (no error)=w390) -> (queue out=w388:refnum<queue>)  [unwired: 2 out]
                n106 = case shown="No Error" w399 {
                  selector: w399 -> [w432 w455]
                  tunnel: w398 -> [w431 w456]
                  tunnel: "Frames" -> [w427 _]
                  tunnel: [w410 w452] -> w386
                  tunnel: w397 -> [w428 _]
                  tunnel: [w409 w454] -> w384
                  tunnel: w395 -> [w426 w450]
                  tunnel: w394 -> [w425 _]
                  tunnel: Stack_Track."Collecting" ("Enum") -> [w424 _]
                  tunnel: [w408 w450] -> _
                  tunnel: w388 -> [w423 _]
                  tunnel: [FALSE ("value") w464] -> w387
                  tunnel: [w407 w453] -> w385
                  frame No Error {
                    w415 = 1 items=["Snap", "Sequence"] ("Capture mode")
                    n107 = call <userlib>:"tm_startcapture_b.vi"("error in (no error)"=w432, "Handle in"=w431) -> ("error out"=w429:errorcluster, "Handle out"=w430:u32)  [unwired: 8 in]
                    n108 = for {
                      N: w427 -> [_]
                      tunnel: w430 -> [w449]
                      tunnel: w429 -> [w448]
                      tunnel: w428 -> [w445]
                      tunnel: [w444] -> w421
                      tunnel: [w443] -> w420
                      tunnel: w426 -> [w441]
                      tunnel: w424 -> [w439]
                      tunnel: w425 -> [w437]
                      tunnel: [w436] -> w414
                      tunnel: w423 -> [w435]
                      i -> [w438]
                      n109 = Bundle By Name(cluster=w437, "Enum"=w439, "Stack Number"=w438) -> (w440:T3)
                      n110 = Enqueue Element(queue=w441, element=w440) -> (queue out=w436:refnum<queue>, error out=w433:errorcluster)  [unwired: 2 in, 1 out]
                      n111 = call <userlib>:"tm_waitnextframe.vi"("error in (no error)"=w448, "Handle in"=w449) -> ("error out"=w446:errorcluster, "Frame Index"=→"Frame Index":i32, "Handle out"=w447:u32)  [unwired: 6 in, 1 out]
                      n112 = call <userlib>:"tm_getframe_a.vi"("error in (no error)"=w446, "Frame Index"=w438, "Buffer Info"=w445, "Handle in"=w447) -> ("error out"=w443:errorcluster, "Data 16"=w434:u16[][], "Handle out"=w444:u32)  [unwired: 3 in, 2 out]
                      n113 = Enqueue Element(queue=w435, element=w434, error in (no error)=w433) -> ()  [unwired: 1 in, 3 out]
                    }
                    n114 = call <userlib>:"tm_stopcapture.vi"("error in (no error)"=w420, "Handle in"=w421) -> ("error out"=w418:errorcluster, "Handle out"=w419:u32)  [unwired: 8 in]
                    n115 = call <userlib>:"tm_unpreparecapture.vi"("error in (no error)"=w418, "Handle in"=w419) -> ("error out"=w417:errorcluster, "Handle out"=w416:u32)  [unwired: 8 in]
                    n116 = Enqueue Element(queue=w414, element=T3 {"Enum"=enum."End", "Stack Number"=0} ("input cluster")) -> (queue out=w408:refnum<queue>)  [unwired: 2 in, 2 out]
                    n117 = call <userlib>:"tm_preparecapture.vi"("error in (no error)"=w417, "Capture mode"=w415, "Handle in"=w416) -> ("error out"=w412:errorcluster, "Buffer Info"=w407:T6, "Handle out"=w411:u32)  [unwired: 5 in, 1 out]
                    n118 = call <userlib>:"tm_startcapture_b.vi"("error in (no error)"=w412, "Handle in"=w411) -> ("error out"=w409:errorcluster, "Handle out"=w410:u32)  [unwired: 8 in]
                  }
                  frame Error {
                    w459 = 1 items=["Snap", "Sequence"] ("Capture mode")
                    # "Prepare camera failure, likely too many frames in stack"
                    n119 = One Button Dialog(message="Too many frames in stack", button name ("OK")="OK") -> (true=w464:bool)
                    n120 = call <userlib>:"tm_stopcapture.vi"("error in (no error)"=w455, "Handle in"=w456) -> ("error out"=w462:errorcluster, "Handle out"=w463:u32)  [unwired: 8 in]
                    n121 = call <userlib>:"tm_unpreparecapture.vi"("error in (no error)"=w462, "Handle in"=w463) -> ("error out"=w461:errorcluster, "Handle out"=w460:u32)  [unwired: 8 in]
                    n122 = Enqueue Element(queue=w450, element=T3 {"Enum"=enum."STOP", "Stack Number"=0} ("input cluster")) -> ()  [unwired: 2 in, 3 out]
                    n123 = call <userlib>:"tm_preparecapture.vi"("error in (no error)"=w461, "Capture mode"=w459, "Handle in"=w460) -> ("error out"=w458:errorcluster, "Buffer Info"=w453:T6, "Handle out"=w457:u32)  [unwired: 5 in, 1 out]
                    n124 = call <userlib>:"tm_startcapture_b.vi"("error in (no error)"=w458, "Handle in"=w457) -> ("error out"=w454:errorcluster, "Handle out"=w452:u32)  [unwired: 8 in]
                  }
                }
              }
            }
          }
          event "HardDisk Record": Value Change {
            n125 = event-data() -> ()  [unwired: 1 in, 5 out]
            n126 = case shown="True" "HardDisk Record" {
              tunnel: w480 -> [w483 w499]
              tunnel: w479 -> [w482 w496]
              tunnel: [w483 w486] -> w478
              tunnel: [w482 w488] -> w477
              tunnel: [w481 w487] -> w473
              tunnel: w472 -> [w481 _]
              tunnel: w470 -> [_ w484]
              tunnel: w469 -> [_ _]
              tunnel: [_ w489] -> w468
              frame False {
              }
              frame True {
                w493 = 0 items=["Snap", "Sequence"] ("Capture mode")
                # "Max 50"
                n127 = call <userlib>:"tm_stopcapture.vi"("error in (no error)"=w499, "Handle in"=w496) -> ("error out"=w498:errorcluster, "Handle out"=w497:u32)  [unwired: 8 in]
                n128 = call <userlib>:"tm_unpreparecapture.vi"("error in (no error)"=w498, "Handle in"=w497) -> ("error out"=w494:errorcluster, "Handle out"=w495:u32)  [unwired: 8 in]
                n129 = call <userlib>:"tm_preparecapture.vi"("error in (no error)"=w494, "Frames"="Frames", "Capture mode"=w493, "Handle in"=w495) -> ("error out"=w492:errorcluster, "Buffer Info"=w490:T6, "Handle out"=w491:u32)  [unwired: 4 in, 1 out]
                "error out 2" <- w492
                n130 = case shown="No Error" w492 {
                  selector: w492 -> [w521 w534]
                  tunnel: w491 -> [w507 w535]
                  tunnel: [w510 w531] -> w488
                  tunnel: w490 -> [w518 _]
                  tunnel: [w509 w533] -> w486
                  tunnel: [FALSE ("value") w543] -> w489
                  tunnel: [w508 w532] -> w487
                  tunnel: "Frames" -> [w504 _]
                  tunnel: w484 -> [_ w529]
                  frame No Error {
                    w513 = 1 items=["Snap", "Sequence"] ("Capture mode")
                    n131 = call <userlib>:"tm_startrecorder.vi"("frames"=w504, "File"="Temp", "Handle in"=w507) -> ("Handle out"=w506:u32)  [unwired: 7 in, 1 out]
                    n132 = call <userlib>:"tm_startcapture_b.vi"("error in (no error)"=w521, "Handle in"=w506) -> ("error out"=w519:errorcluster, "Handle out"=w520:u32)  [unwired: 8 in]
                    n133 = while {
                      tunnel: w520 -> [w527]
                      tunnel: w519 -> [w526]
                      tunnel: w518 -> [_]
                      tunnel: [w528] -> w516
                      tunnel: w504 -> [w523]
                      stop <- w524 stop-if-true
                      n134 = Wait (ms)(milliseconds to wait=u32 50) -> ()  [unwired: 1 out]
                      n135 = call <userlib>:"tm_getrecorderstatus.vi"("error in (no error)"=w526, "Handle"=w527) -> ("error out"=w528:errorcluster, "Count"=w522:i32)  [unwired: 6 in, 2 out]
                      "Count" <- w522
                      n136 = Equal?(x=w522, y=w523) -> (x = y?=w524:bool)
                    }
                    n137 = call <userlib>:"tm_stopcapture.vi"("error in (no error)"=w516) -> ("error out"=w503:errorcluster, "Handle out"=w501:u32)  [unwired: 9 in]
                    n138 = call <userlib>:"tm_stoprecorder.vi"("error in (no error)"=w503, "Handle in"=w501) -> ("error out"=w502:errorcluster, "Handle out"=w500:u32)  [unwired: 8 in]
                    n139 = call <userlib>:"tm_unpreparecapture.vi"("error in (no error)"=w502, "Handle in"=w500) -> ("error out"=w515:errorcluster, "Handle out"=w514:u32)  [unwired: 8 in]
                    n140 = call <userlib>:"tm_preparecapture.vi"("error in (no error)"=w515, "Capture mode"=w513, "Handle in"=w514) -> ("error out"=w512:errorcluster, "Buffer Info"=w508:T6, "Handle out"=w511:u32)  [unwired: 5 in, 1 out]
                    n141 = call <userlib>:"tm_startcapture_b.vi"("error in (no error)"=w512, "Handle in"=w511) -> ("error out"=w509:errorcluster, "Handle out"=w510:u32)  [unwired: 8 in]
                  }
                  frame Error {
                    w538 = 1 items=["Snap", "Sequence"] ("Capture mode")
                    # "Prepare camera failure, likely too many frames in stack"
                    n142 = One Button Dialog(message="Too many frames in stack", button name ("OK")="OK") -> (true=w543:bool)
                    n143 = call <userlib>:"tm_stopcapture.vi"("error in (no error)"=w534, "Handle in"=w535) -> ("error out"=w541:errorcluster, "Handle out"=w542:u32)  [unwired: 8 in]
                    n144 = call <userlib>:"tm_unpreparecapture.vi"("error in (no error)"=w541, "Handle in"=w542) -> ("error out"=w540:errorcluster, "Handle out"=w539:u32)  [unwired: 8 in]
                    n145 = Enqueue Element(queue=w529, element=T3 {"Enum"=enum."STOP", "Stack Number"=0} ("input cluster")) -> ()  [unwired: 2 in, 3 out]
                    n146 = call <userlib>:"tm_preparecapture.vi"("error in (no error)"=w540, "Capture mode"=w538, "Handle in"=w539) -> ("error out"=w537:errorcluster, "Buffer Info"=w532:T6, "Handle out"=w536:u32)  [unwired: 5 in, 1 out]
                    n147 = call <userlib>:"tm_startcapture_b.vi"("error in (no error)"=w537, "Handle in"=w536) -> ("error out"=w533:errorcluster, "Handle out"=w531:u32)  [unwired: 8 in]
                  }
                }
              }
            }
          }
          event "Scan Mode": Value Change {
            w546 = u32 4211872 items=["SENSOR MODE"=4212128, "CCD MODE"=4212384, "READOUT MODE"=4211872, "ACTIVE VIEW INDEX"=4343136, "BITS PER CHANNEL"=4342976, "IMAGE PIXEL TYPE"=4343296, "BINNING"=4215968, "EXPOSURE TIME"=2049184, "CONTRAST GAIN"=3163312, "CONTRAST OFFSET"=3163328, "LIGHT MODE"=2114720, "SENSITIVITY"=2114992, "PHOTON IMAGING MODE"=2115200, "HIGH DYNAMIC RANGE MODE"=3163360, "WHITE BALANCE"=3163568, "TEMPERATURE"=2115232, "TEMPERATURE TARGET"=2115264, "SENSOR COOLER FAN"=2115296, "LINEBUNDLE HEIGHT"=4212192, "MECHANICAL SHUTTER"=2115488, "BACK FOCUS POSITION"=8422304, "TRIGGER CONNECTOR"=1066432, "TRIGGER SOURCE"=1066144, "OUTPUT TRIGGER SOURCE"=1852576, "TRIGGER GLOBAL EXPOSURE"=2049680, "FIRST TRIGGER BEHAVIOR"=2049696, "CHANNEL SYNC"=1852352, "READOUT DIRECTION"=4211904, "PRE HSYNC COUNT"=1852704] ("Parameter")
            w561 = 1 items=["Snap", "Sequence"] ("Capture mode")
            n148 = event-data() -> ("NewVal"=w551:dbl)  [unwired: 1 in, 2 out]
            n149 = call <userlib>:"tm_stopcapture.vi"("error in (no error)"=w562, "Handle in"=w563) -> ("error out"=w564:errorcluster, "Handle out"=w565:u32)  [unwired: 8 in]
            n150 = call <userlib>:"tm_unpreparecapture.vi"("error in (no error)"=w564, "Handle in"=w565) -> ("error out"=w549:errorcluster, "Handle out"=w550:u32)  [unwired: 8 in]
            n151 = call <userlib>:"tm_setparameter_a.vi"("error in (no error)"=w549, "Value in"=w551, "Parameter"=w546, "Handle in"=w550) -> ("error out"=w548:errorcluster, "Handle out"=w547:u32)  [unwired: 6 in]
            n152 = call <userlib>:"tm_getparameter_a.vi"("error in (no error)"=w548, "Parameter"=w546, "Handle in"=w547) -> ("error out"=w554:errorcluster, "Value out"=w553:dbl, "Handle out"=w552:u32)  [unwired: 6 in]
            n153 = local write "SMD"(w553) -> ()
            n154 = call <userlib>:"tm_preparecapture.vi"("error in (no error)"=w554, "Capture mode"=w561, "Handle in"=w552) -> ("error out"=w559:errorcluster, "Buffer Info"=w556:T6, "Handle out"=w560:u32)  [unwired: 5 in, 1 out]
            n155 = call <userlib>:"tm_startcapture_b.vi"("error in (no error)"=w559, "Handle in"=w560) -> ("error out"=w558:errorcluster, "Handle out"=w557:u32)  [unwired: 8 in]
          }
          event "Binning": Value Change {
            w570 = u32 4215968 items=["BINNING"=4215968, "BITS PER CHANNEL"=2, "ACTIVE VIEW INDEX"=3, "CCD MODE"=4, "SENSOR MODE"=5, "READOUT MODE"=6, "EXPOSURE TIME"=7, "CONTRAST GAIN"=8, "CONTRAST OFFSET"=9, "LIGHT MODE"=10, "SENSITIVITY"=11, "WHITE BALANCE"=12, "PHOTON IMAGING MODE"=13, "HIGH DYNAMIC RANGE MODE"=14, "TRIGGER SOURCE"=15, "TRIGGER ACTIVE"=16, "TRIGGER MODE"=17, "TRIGGER POLARITY"=18, "TRIGGER GLOBAL EXPOSURE"=19, "FIRST TRIGGER BEHAVIOR"=20, "TRIGGER TIMES"=21, "OUTPUT TRIGGER POLARITY"=22, "OUTPUT TRIGGER DELAY"=23, "OUTPUT TRIGGER PERIOD"=24, "TEMPERATURE"=25, "TEMPERATURE TARGET"=26, "SENSOR COOLER FAN"=27, "MECHANICAL SHUTTER"=28, "BACK FOCUS POSITION"=29, "FRAMEBUNDLE MODE"=30, "FRAMEBUNDLE NUMBER"=31, "LINEBUNDLE HEIGHT"=32, "TRIGGER CONNECTOR"=33, "IMAGE PIXEL TYPE"=34, "OUTPUT TRIGGER KIND"=35, "READOUT DIRECTION"=36, "CHANNEL SYNC"=37] ("Parameter")
            w609 = 1 items=["Snap", "Sequence"] ("Capture mode")
            n156 = event-data() -> ("NewVal"=w571:u16)  [unwired: 1 in, 2 out]
            n157 = call <userlib>:"tm_stopcapture.vi"("error in (no error)"=w578, "Handle in"=w579) -> ("error out"=w576:errorcluster, "Handle out"=w577:u32)  [unwired: 8 in]
            n158 = call <userlib>:"tm_unpreparecapture.vi"("error in (no error)"=w576, "Handle in"=w577) -> ("error out"=w572:errorcluster, "Handle out"=w569:u32)  [unwired: 8 in]
            n159 = call <userlib>:"tm_setparameter_a.vi"("error in (no error)"=w572, "Value in"=w571, "Parameter"=w570, "Handle in"=w569) -> ("error out"=w573:errorcluster, "Handle out"=w574:u32)  [unwired: 6 in]
            n160 = call <userlib>:"tm_getarea_a.vi"("error in (no error)"=w573, "Handle in"=w574) -> ("error out"=w597:errorcluster, "V Offset"=w599:T5, "H Offset"=w598:T5, "Handle out"=w596:u32, "H Width"=w600:T5, "V Width"=w601:T5)  [unwired: 4 in]
            n161 = Unbundle By Name(w598) -> ("Value"=w592:i32, "Minimum"=w595:i32, "Maximum"=w594:i32, "Increment"=w593:i32)
            n162 = Unbundle By Name(w599) -> ("Value"=w582:i32, "Minimum"=w591:i32, "Maximum"=w590:i32, "Increment"=w589:i32)
            n163 = Unbundle By Name(w600) -> ("Value"=w581:i32, "Minimum"=w588:i32, "Maximum"=w587:i32, "Increment"=w586:i32)
            n164 = Unbundle By Name(w601) -> ("Value"=w580:i32, "Minimum"=w585:i32, "Maximum"=w584:i32, "Increment"=w583:i32)
            n165 = property on="H Offset" class="DigNum (strict)"("Value"=w592, "Minimum"=w595, "Maximum"=w594, "Increment"=w593) -> ()  [unwired: 2 in, 2 out]
            n166 = property on="V Offset" class="DigNum (strict)"("Value"=w582, "Minimum"=w591, "Maximum"=w590, "Increment"=w589) -> ()  [unwired: 2 in, 2 out]
            n167 = property on="H Width" class="DigNum (strict)"("Value"=w581, "Minimum"=w588, "Maximum"=w587, "Increment"=w586) -> ()  [unwired: 2 in, 2 out]
            n168 = property on="V Width" class="DigNum (strict)"("Value"=w580, "Minimum"=w585, "Maximum"=w584, "Increment"=w583) -> ()  [unwired: 2 in, 2 out]
            n169 = local write "SHO"(w592) -> ()
            n170 = local write "SVO"(w582) -> ()
            n171 = local write "SHW"(w581) -> ()
            n172 = local write "SVW"(w580) -> ()
            n173 = call <userlib>:"tm_preparecapture.vi"("error in (no error)"=w597, "Capture mode"=w609, "Handle in"=w596) -> ("error out"=w607:errorcluster, "Buffer Info"=w604:T6, "Handle out"=w608:u32)  [unwired: 5 in, 1 out]
            n174 = call <userlib>:"tm_startcapture_b.vi"("error in (no error)"=w607, "Handle in"=w608) -> ("error out"=w606:errorcluster, "Handle out"=w605:u32)  [unwired: 8 in]
          }
          event "H Offset", "H Width", "V Offset", "V Width": Value Change {
            w654 = 1 items=["Snap", "Sequence"] ("Capture mode")
            n175 = event-data() -> ()  [unwired: 1 in, 4 out]
            n176 = call <userlib>:"tm_stopcapture.vi"("error in (no error)"=w616, "Handle in"=w617) -> ("error out"=w614:errorcluster, "Handle out"=w615:u32)  [unwired: 8 in]
            n177 = local read "H Offset"() -> (w620:i32)
            n178 = local read "H Width"() -> (w621:i32)
            n179 = local read "V Offset"() -> (w622:i32)
            n180 = local read "V Width"() -> (w619:i32)
            n181 = call <userlib>:"tm_unpreparecapture.vi"("error in (no error)"=w614, "Handle in"=w615) -> ("error out"=w612:errorcluster, "Handle out"=w613:u32)  [unwired: 8 in]
            n182 = Bundle("H Offset"=w620, "V Offset"=w622, "H Width"=w621, "V Width"=w619) -> (w618:T7)  [unwired: 1 in]
            n183 = call <userlib>:"tm_setarea.vi"("error in (no error)"=w612, "Sub Region"=w618, "Handle in"=w613) -> ("error out"=w623:errorcluster, "Handle out"=w624:u32)  [unwired: 7 in]
            n184 = call <userlib>:"tm_getarea_a.vi"("error in (no error)"=w623, "Handle in"=w624) -> ("error out"=w642:errorcluster, "V Offset"=w644:T5, "H Offset"=w643:T5, "Handle out"=w641:u32, "H Width"=w645:T5, "V Width"=w646:T5)  [unwired: 4 in]
            n185 = Unbundle By Name(w643) -> ("Value"=w637:i32, "Minimum"=w640:i32, "Maximum"=w639:i32, "Increment"=w638:i32)
            n186 = Unbundle By Name(w644) -> ("Value"=w627:i32, "Minimum"=w636:i32, "Maximum"=w635:i32, "Increment"=w634:i32)
            n187 = Unbundle By Name(w645) -> ("Value"=w626:i32, "Minimum"=w633:i32, "Maximum"=w632:i32, "Increment"=w631:i32)
            n188 = Unbundle By Name(w646) -> ("Value"=w625:i32, "Minimum"=w630:i32, "Maximum"=w629:i32, "Increment"=w628:i32)
            n189 = property on="H Offset" class="DigNum (strict)"("Value"=w637, "Minimum"=w640, "Maximum"=w639, "Increment"=w638) -> ()  [unwired: 2 in, 2 out]
            n190 = property on="V Offset" class="DigNum (strict)"("Value"=w627, "Minimum"=w636, "Maximum"=w635, "Increment"=w634) -> ()  [unwired: 2 in, 2 out]
            n191 = property on="H Width" class="DigNum (strict)"("Value"=w626, "Minimum"=w633, "Maximum"=w632, "Increment"=w631) -> ()  [unwired: 2 in, 2 out]
            n192 = property on="V Width" class="DigNum (strict)"("Value"=w625, "Minimum"=w630, "Maximum"=w629, "Increment"=w628) -> ()  [unwired: 2 in, 2 out]
            n193 = local write "SHO"(w637) -> ()
            n194 = local write "SVO"(w627) -> ()
            n195 = local write "SHW"(w626) -> ()
            n196 = local write "SVW"(w625) -> ()
            n197 = call <userlib>:"tm_preparecapture.vi"("error in (no error)"=w642, "Capture mode"=w654, "Handle in"=w641) -> ("error out"=w652:errorcluster, "Buffer Info"=w649:T6, "Handle out"=w653:u32)  [unwired: 5 in, 1 out]
            n198 = call <userlib>:"tm_startcapture_b.vi"("error in (no error)"=w652, "Handle in"=w653) -> ("error out"=w651:errorcluster, "Handle out"=w650:u32)  [unwired: 8 in]
          }
        }
        n199 = Unbundle By Name(w172) -> ("status"=w185:bool)
        n200 = Compound Arithmetic op=OR(w185, "stop", w163) -> (w184:bool)
      }
      n201 = while {
        tunnel: w29 -> [w109]
        shift-right: [w105] -> _
        shift-left: _ -> [w103]
        shift-right: [w101] -> _
        shift-left: _ -> [w102]
        tunnel: w30 -> [w99]
        shift-right: [w97] -> _
        shift-left: _ -> [w96]
        stop <- w104 stop-if-true
        n202 = Dequeue Element(queue=w109, timeout in ms (-1)=1) -> (element=w108:T3)  [unwired: 1 in, 3 out]
        n203 = Unbundle By Name(w108) -> ("Enum"=w107:T1, "Stack Number"=w106:i32)
        "Enum" <- w107
        n204 = Dequeue Element(queue=w99) -> (element=w95:u16[][], timed out?=w98:bool)  [unwired: 2 in, 2 out]
        n205 = case shown="False" w98 {
          tunnel: w95 -> [w111 w113]
          tunnel: [w111 w112] -> w93
          tunnel: [w110 w113] -> w97
          tunnel: w96 -> [w110 w112]
          frame False {
          }
          frame True {
          }
        }
        "Image" <- w93
        n206 = case shown="\"Start Sequence\"" w107 {
          tunnel: w106 -> [_ w131 _ _ _]
          tunnel: [w123 w141 w157 _ _] -> w105
          tunnel: w103 -> [_ w144 w157 _ _]
          tunnel: [FALSE _ _ TRUE _] -> w104
          tunnel: w93 -> [_ w143 _ _ _]
          tunnel: w102 -> [w121 w139 w155 w158 w160]
          tunnel: [w122 w138 w154 w158 w160] -> w101
          tunnel: "Path" -> [w117 _ _ _ _]
          frame "Start Sequence" {
            # "Public tiff library"
            # "Get path and open file"
            n207 = Equal?(x=w117, y=path "") -> (x = y?=w119:bool)
            n208 = case shown="True" w119 {
              tunnel: w117 -> [w124 _]
              tunnel: [w124 w127] -> w116
              frame False {
              }
              frame True {
                n209 = call "File Dialog"("pattern (all files)"=".tiff", "pattern label"="Tiff Image") -> ("selected path"=w127:path)  [unwired: 10 in, 3 out]
              }
            }
            n210 = case shown="False" "AutoIncrement" {
              tunnel: w116 -> [w128 w130]
              tunnel: [w128 w129] -> w115
              frame False {
              }
              frame True {
                n211 = call "4Digit File Incrementer.vi"("path"=w130) -> ("appended path"=w129:path)  [unwired: 10 in]
              }
            }
            n212 = call "libtiff2_open_w.vi"("error in (no error)"=w121, "Input path"=w115) -> ("error out"=w122:errorcluster, "handle"=w123:i32)  [unwired: 8 in]
            n213 = local write "Path"(w115) -> ()
          }
          frame "Collecting" {
            w147 = T8 7 items=["Grayscale (U8)", "Grayscale (I16)", "Grayscale (SGL)", "Complex (CSG)", "RGB (U32)", "HSL (U32)", "RGB (U64)", "Grayscale (U16)"] ("Image Type")
            # "Add Image to write scan line"
            n214 = Number To Decimal String(number=w131) -> (decimal integer string=w132:string)  [unwired: 1 in]
            n215 = call "IMAQ Create"("Image Name"="Sim Stack", "Image Type"=w147) -> ("New Image"=w136:T9)  [unwired: 3 in, 1 out]
            n216 = call "IMAQ Write Custom Data"("Custom Data In"=w132, "Key"="test", "Image"=w136) -> ("error out"=w134:errorcluster, "Image Out"=w135:T9)  [unwired: 7 in]
            n217 = call "IMAQ ArrayToImage"("Image Pixels (U16)"=w143, "error in (no error)"=w134, "Image"=w135) -> ("Image Out"=w145:T9)  [unwired: 7 in, 1 out]
            n218 = call "libtiff2_writeScanLine_U16.vi"("error in (no error)"=w139, "page"=w131, "Image"=w145, "Handle"=w144) -> ("error out"=w142:errorcluster, "Handle out"=w141:i32)  [unwired: 6 in]
            n219 = case shown="Error" w142 {
              selector: w142 -> [w148 w150]
              tunnel: w141 -> [_ w151]
              tunnel: [w148 w149] -> w138
              frame No Error {
              }
              frame Error {
                n220 = call "libtiff2_close.vi"("error in (no error)"=w150, "Handle"=w151) -> ("error out"=w149:errorcluster)  [unwired: 8 in]
              }
            }
            n221 = property on="Capture" class="Bool (strict)"("DisabledEnum"=T2."Disabled and Grayed Out" ("Disabled"), "BoolText.Text"="Saving" ("Boolean Text.Text")) -> ()  [unwired: 2 in, 2 out]
          }
          frame "End" {
            (unwired) FALSE
            # "Close image file, reset capturing button"
            n222 = call "libtiff2_close.vi"("error in (no error)"=w155, "Handle"=w157) -> ("error out"=w156:errorcluster)  [unwired: 8 in]
            n223 = property on="Capture" class="Bool (strict)"(error in=w156, "BoolText.Text"="OK" ("Boolean Text.Text"), "DisabledEnum"=T2."Enabled" ("Disabled")) -> (error out=w154:errorcluster)  [unwired: 1 in, 1 out]
          }
          frame "STOP" {
          }
          frame "Idle" {
          }
        }
      }
      n224 = call <userlib>:"tm_stopcapture.vi"("error in (no error)"=w60, "Handle in"=w61) -> ("error out"=w57:errorcluster, "Handle out"=w58:u32)  [unwired: 8 in]
      n225 = call <userlib>:"tm_unpreparecapture.vi"("error in (no error)"=w57, "Handle in"=w58) -> ("error out"=w56:errorcluster, "Handle out"=w59:u32)  [unwired: 8 in]
      n226 = call <userlib>:"tm_closecamera.vi"("error in (no error)"=w56, "Handle in"=w59) -> ("error out"=w90:errorcluster)  [unwired: 9 in]
      n227 = call <userlib>:"tm_deinitialize.vi"("error in (no error)"=w90) -> ("error out"=w89:errorcluster)  [unwired: 10 in]
    }
  }
  "error out" <- w3
